vi "XIPIN_AXI_Quad_SPI_3_2.vi"   [LabVIEW 2017]
doc: "SPI Interface for SPI Based Slave\n------------------------------------\n<b>Need License</b> : No\n<b>Interface</b> : AXI4"
uses:
  <vilib>/rvi/XilinxIP/XIPIN_XNode/niFpgaXIPIN.xnode
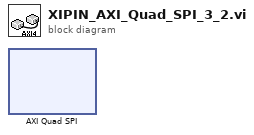
[diagram p0: block diagram]
diagram:
  n1 = xnode ("AXI Quad SPI")() -> ()
